vi "Setup servo out.vi"(8 "error in (no error)":errorcluster, 10 "signal":waveform(dbl), 11 "Sampling info in":T1={"Channels"=[], "Sampling freq"=0.0, "Output freq"=0.0, "Update freq"=0.0, "Steps per rev"=0, "Counts per rev"=0, "Amplifier"="", "Motor driver"="", "Step bit"=0, "Max speed"=0.0, "Max accel"=0.0, "Pos gain"=0.0, "Vel gain"=0.0, "counter"="Dev1/ctr0"} {"Channels"."Hi cutoff" items=["500"=500.0, "1k"=1000.0, "5k"=5000.0, "10k"=10000.0, "20k"=20000.0]; "Channels"."Lo cutoff" items=["0.1"=0.1, "1"=1.0, "10"=10.0, "100"=100.0, "300"=300.0]; "Channels"."Gain" items=["x100"=100, "x1000"=1000, "x10000"=10000]}) -> (0 "error out":errorcluster, 2 "task out":refnum<k21>, 4 "compensated":dbl[](array[numeric]))   [LabVIEW 2013]
uses:
  Sampling info.ctl
  Channel.ctl
  <vilib>/DAQmx/write.llb/DAQmx Write (Counter 1D Frequency 1Chan NSamp).vi
  <vilib>/DAQmx/create/channels.llb/DAQmx Create Channel (CO-Pulse Generation-Frequency).vi
  <vilib>/DAQmx/configure/timing.llb/DAQmx Timing (Implicit).vi
  <vilib>/DAQmx/miscellaneous.llb/DAQmx Fill In Error Info.vi
panel:
  out "number of samples written":u32
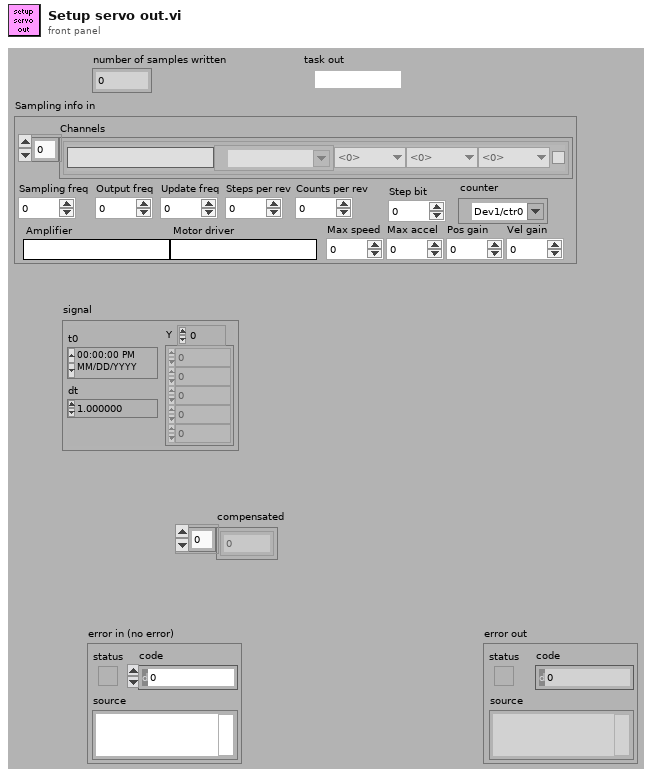
[diagram p1: front panel]
types:
  T1 = typedef "Sampling info.ctl" = cluster{"Channels":T2[], "Sampling freq":dbl, "Output freq":dbl, "Update freq":dbl, "Steps per rev":i32, "Counts per rev":i32, "Amplifier":string, "Motor driver":string, "Step bit":u8, "Max speed":dbl, "Max accel":dbl, "Pos gain":dbl, "Vel gain":dbl, "counter":tag}
  T2 = typedef "Channel.ctl" = cluster{"Name":string, "Chan":tag, "Gain":u32, "Lo cutoff":dbl, "Hi cutoff":dbl, "Notch":bool}
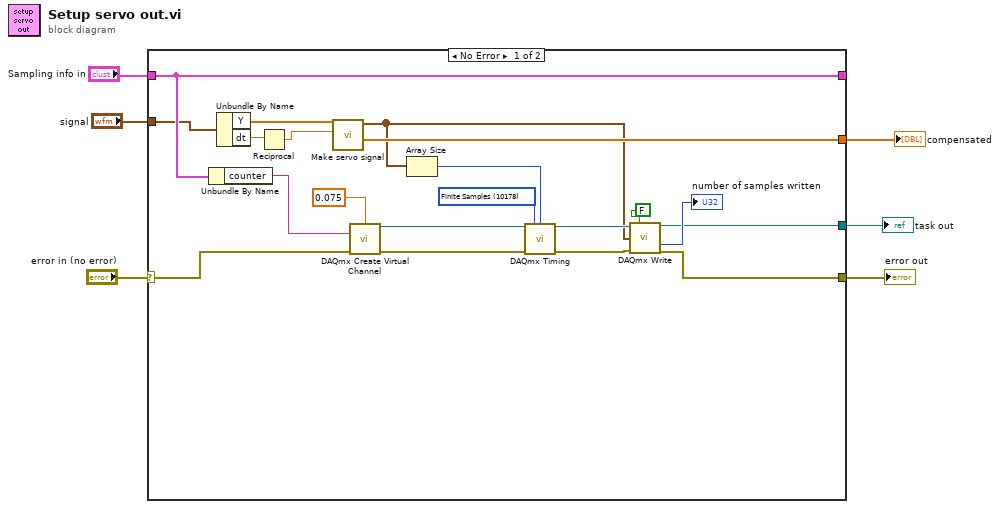
[diagram p0: block diagram]
diagram:
  n1 = case shown="No Error" "error in (no error)" {
    selector: "error in (no error)" -> [w22 w27]
    tunnel: [w25 w27] -> w5
    tunnel: [w24 w28] -> _
    tunnel: "Sampling info in" -> [w24 w28]
    tunnel: [w16 _] -> w3
    tunnel: "signal" -> [w15 _]
    tunnel: [w14 _] -> w1
    frame No Error {
      w19 = 10178 items=["Finite Samples"=10178, "Continuous Samples"=10123, "Hardware Timed Single Point"=12522] ("sample mode")
      n2 = Unbundle By Name(w24) -> ("counter"=w20:tag)
      n3 = Unbundle By Name(w15) -> ("Y"=w9:dbl[], "dt"=w8:dbl)
      n4 = Reciprocal(x=w8) -> (1/x=w7:dbl)
      n5 = call "Make servo signal.vi"("sampling frequency"=w7, "Data"=w9) -> ("compensated"=w14:dbl[], "sine PWM pattern"=w11:cluster{"duty cycle":dbl, "frequency":dbl}[])  [unwired: 7 in, 1 out]
      n6 = call-poly <vilib>:"DAQmx Create Virtual Channel.vi"("duty cycle"=0.075, "counter"=w20, "error in"=w22) -> ("task out"=w23:refnum<k21>, "error out"=w21:errorcluster)  [unwired: 11 in]
      n7 = Array Size(array=w11) -> (size(s)=w10:i32)
      n8 = call-poly <vilib>:"DAQmx Timing.vi"("task/channels in"=w23, "sample mode"=w19, "samples per channel"=w10, "error in"=w21) -> ("task out"=w13:refnum<k21>, "error out"=w12:errorcluster)  [unwired: 10 in]
      n9 = call-poly <vilib>:"DAQmx Write.vi"("task/channels in"=w13, "auto start"=FALSE, "data"=w11, "error in"=w12) -> ("task out"=w16:refnum<k21>, "number of samples written per channel"=→"number of samples written":u32, "error out"=w25:errorcluster)  [unwired: 9 in]
    }
    frame Error {
    }
  }
  "error out" <- w5
  "task out" <- w3
  "compensated" <- w1
